vi "Team and Side.vi"(5 "Lado":enum16{"Esquerdo", "Direito"}(ring) caption="Enum", 7 "Time":enum16{"Azul", "Amarelo"}(ring) caption="Enum", 8 "Enemy state and balls":T2, 9 "IA_State":T12, 10 "Game Status":T18 {"Time" format="%<%.3X %x>T"; "Blue Timeout Remaining" format="%<%M:%S>t"; "Yellow Timeout Remaining" format="%<%M:%S>t"; "Time Left" format="%<%M:%S>t"}, 11 "Field State Input":T13 {"Detection Frame Out"."robots_blue"."height" format="%+4.3f"; "Detection Frame Out"."robots_blue"."pixel_y" format="%+4.3f"; "Detection Frame Out"."robots_blue"."pixel_x" format="%+4.3f"; "Detection Frame Out"."robots_blue"."orientation" format="%+4.3f"; "Detection Frame Out"."robots_blue"."y" format="%+4.3f"; "Detection Frame Out"."robots_blue"."confidence" format="%4.3f"; "Detection Frame Out"."robots_blue"."x" format="%+4.3f"; "Detection Frame Out"."robots_yellow"."height" format="%+4.3f"; "Detection Frame Out"."robots_yellow"."pixel_y" format="%+4.3f"; "Detection Frame Out"."robots_yellow"."pixel_x" format="%+4.3f"; "Detection Frame Out"."robots_yellow"."orientation" format="%+4.3f"; "Detection Frame Out"."robots_yellow"."y" format="%+4.3f"; "Detection Frame Out"."robots_yellow"."confidence" format="%4.3f"; "Detection Frame Out"."robots_yellow"."x" format="%+4.3f"}) -> (3 "IA State":T7={"our_robots"=[], "enemy_robots"=[], "balls"=[], "geometry"={"line_width"=0, "field_length"=0, "field_width"=0, "boundary_width"=0, "referee_width"=0, "goal_width"=0, "goal_depth"=0, "goal_wall_width"=0, "center_circle_radius"=0, "defense_radius"=0, "defense_stretch"=0, "free_kick_from_defense_dist"=0, "penalty_spot_from_field_line_dist"=0, "penalty_line_from_spot_dist"=0}, "IA Judge"={"stage"="", "command"="", "our_goalie_id"=0.0, "enemy_goalie_id"=0.0, "command enum"=enum."Halt", "Time"=enum."Azul"}, "Received Timestamp"=timestamp(0 s since 1904-01-01), "Events"={"Touch"=FALSE, "Ball out"=FALSE, "id touch"=0.0, "Ball out of \nVision"=FALSE, "Ball inside \nGoalie area"=FALSE, "Robot not responding"=FALSE, "Robots responding status"=[1.0, 1.0, 1.0, 1.0, 1.0, 1.0], "Enemy Ball \nPossession"=FALSE, "Pass State"=FALSE, "id end of pass"=0.0, "Kick"=FALSE, "Id ini Possession"=0.0, "Ball Possesion"=FALSE, "Id Possesion"=0.0}})   [LabVIEW 2017]
uses:
  SSL Referee Game Status.ctl
  AI Input.ctl
  AI Robot.ctl
  Intel/Functions Enum.ctl
  Intel/AttackerStates.ctl
  AI Ball.ctl
  Field Size.ctl
  AI Judge.ctl
  Intel/Command Enum.ctl
  Util/Events/Events.ctl
  SSL/SSL Field State.ctl
  SSL Detection Frame.ctl
  SSL Detection Robot.ctl
  <vilib>/Analysis/Matrix/Datatypes/RealMatrix.ctl
  SSL Detection Ball.ctl
  <vilib>/Analysis/Matrix/NI_Matrix.lvlib
panel:
  in  "enemy_robots":T3[](array[typedef])
  in  "?":T6
  in  "?":T6
  in  "output cluster":T7={"our_robots"=[], "enemy_robots"=[], "balls"=[], "geometry"={"line_width"=0, "field_length"=0, "field_width"=0, "boundary_width"=0, "referee_width"=0, "goal_width"=0, "goal_depth"=0, "goal_wall_width"=0, "center_circle_radius"=0, "defense_radius"=0, "defense_stretch"=0, "free_kick_from_defense_dist"=0, "penalty_spot_from_field_line_dist"=0, "penalty_line_from_spot_dist"=0}, "IA Judge"={"stage"="", "command"="", "our_goalie_id"=0.0, "enemy_goalie_id"=0.0, "command enum"=enum."Halt", "Time"=enum."Azul"}, "Received Timestamp"=timestamp(0 s since 1904-01-01), "Events"={"Touch"=FALSE, "Ball out"=FALSE, "id touch"=0.0, "Ball out of \nVision"=FALSE, "Ball inside \nGoalie area"=FALSE, "Robot not responding"=FALSE, "Robots responding status"=[1.0, 1.0, 1.0, 1.0, 1.0, 1.0], "Enemy Ball \nPossession"=FALSE, "Pass State"=FALSE, "id end of pass"=0.0, "Kick"=FALSE, "Id ini Possession"=0.0, "Ball Possesion"=FALSE, "Id Possesion"=0.0}}
  # "Score"
  # "Red Cards"
  # "Yellow Cards"
  # "Timeouts Left"
  # "Timeout Remaining"
  # "Goalie ID"
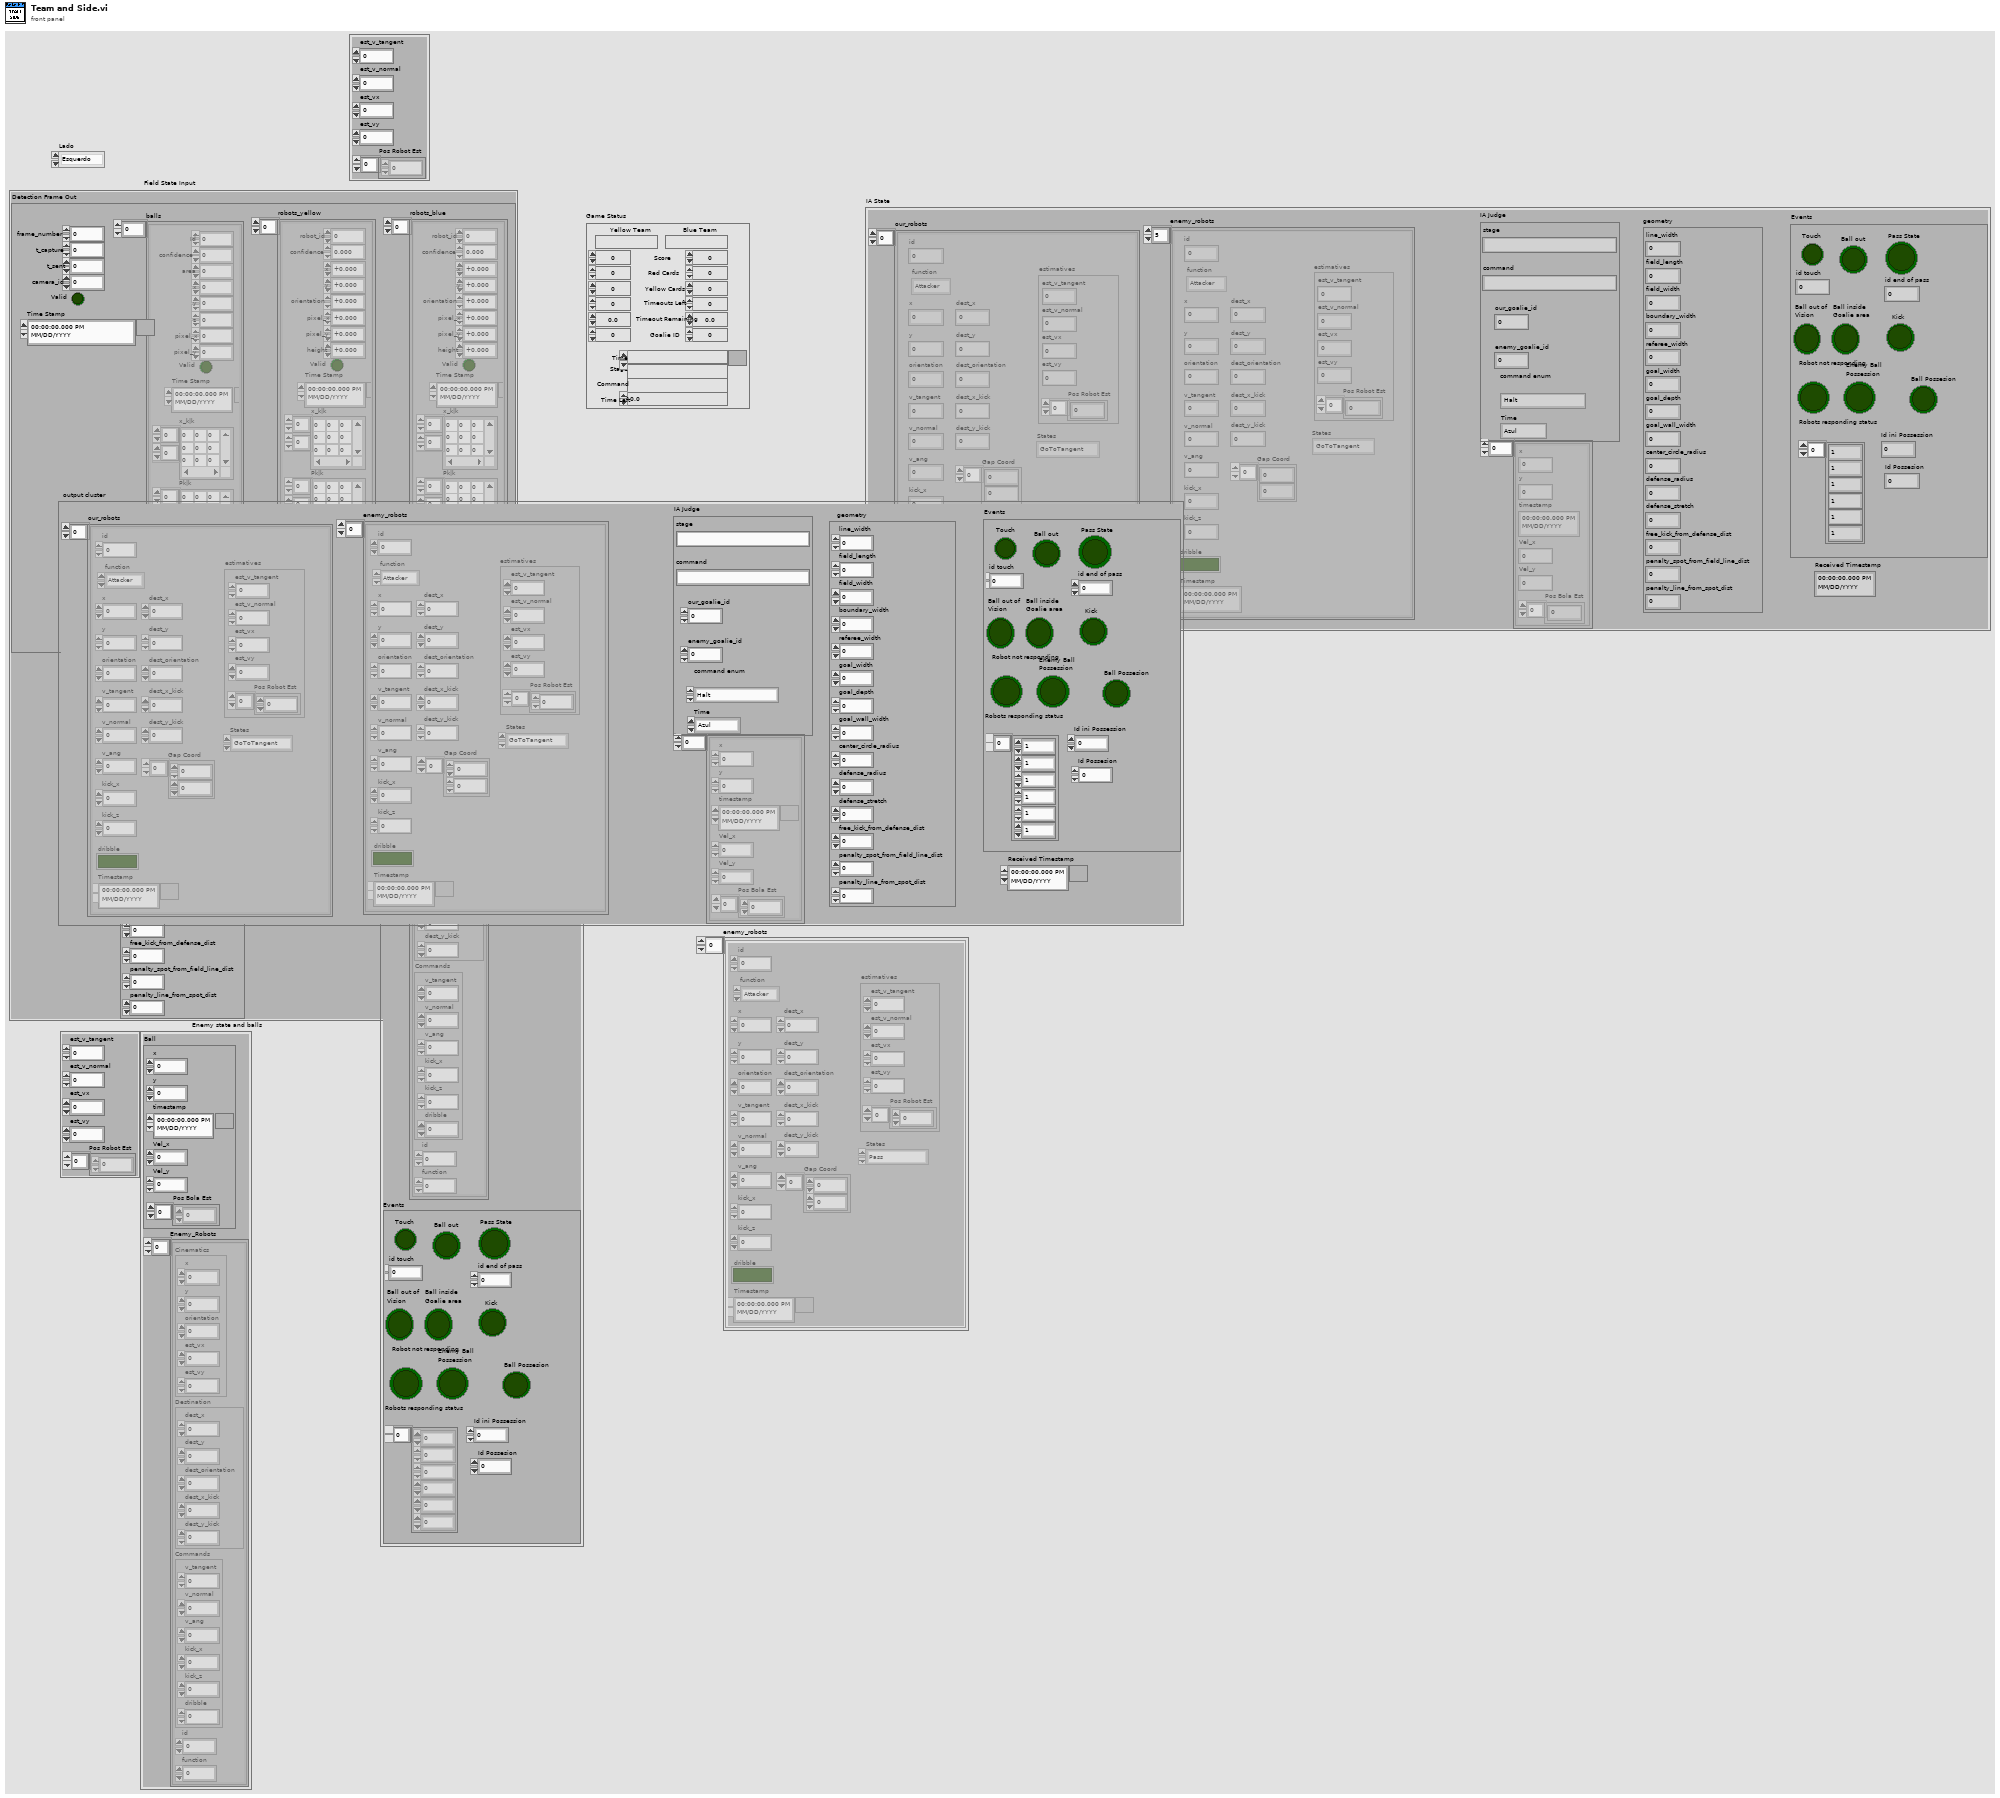
[diagram p1: front panel]
types:
  T1 = typedef "AI Ball.ctl" = cluster{"x":dbl, "y":dbl, "timestamp":timestamp, "Vel_x":dbl, "Vel_y":dbl, "Pos Bola Est":dbl[]}
  T2 = cluster{"Ball":T1, "Enemy_Robots":cluster{"Cinematics":cluster{"x":dbl, "y":dbl, "orientation":dbl, "est_vx":dbl, "est_vy":dbl}, "Destination":cluster{"dest_x":dbl, "dest_y":dbl, "dest_orientation":dbl, "dest_x_kick":dbl, "dest_y_kick":dbl}, "Commands":cluster{"v_tangent":dbl, "v_normal":dbl, "v_ang":dbl, "kick_x":dbl, "kick_z":dbl, "dribble":u32}, "id":u32, "function":u32}[]}
  T3 = typedef "AI Robot.ctl" = cluster{"id":u32, "function":T4, "x":dbl, "y":dbl, "orientation":dbl, "v_tangent":dbl, "v_normal":dbl, "v_ang":dbl, "kick_x":dbl, "kick_z":dbl, "dribble":bool, "Timestamp":timestamp, "dest_x":dbl, "dest_y":dbl, "dest_orientation":dbl, "estimatives":cluster{"est_v_tangent":dbl, "est_v_normal":dbl, "est_vx":dbl, "est_vy":dbl, "Pos Robot Est":dbl[]}, "dest_x_kick":dbl, "dest_y_kick":dbl, "Gap Coord":dbl[], "States":T5}
  T4 = typedef "Functions Enum.ctl" = enum16{"Attacker", "Goalie", "Defender", "Striker", "Goto 0", "Dummy", "Kicker", "ZigZag"}
  T5 = typedef "AttackerStates.ctl" = enum16{"Pass", "GoToTangent", "BallGetting", "GoToKick", ""}
  T6 = cluster{"est_v_tangent":dbl, "est_v_normal":dbl, "est_vx":dbl, "est_vy":dbl, "Pos Robot Est":dbl[]}
  T7 = typedef "AI Input.ctl" = cluster{"our_robots":T3[], "enemy_robots":T3[], "balls":T1[], "geometry":T8, "IA Judge":T9, "Received Timestamp":timestamp, "Events":T11}
  T8 = typedef "Field Size.ctl" = cluster{"line_width":u32, "field_length":u32, "field_width":u32, "boundary_width":u32, "referee_width":u32, "goal_width":u32, "goal_depth":u32, "goal_wall_width":u32, "center_circle_radius":u32, "defense_radius":u32, "defense_stretch":u32, "free_kick_from_defense_dist":u32, "penalty_spot_from_field_line_dist":u32, "penalty_line_from_spot_dist":u32}
  T9 = typedef "AI Judge.ctl" = cluster{"stage":string, "command":string, "our_goalie_id":dbl, "enemy_goalie_id":dbl, "command enum":T10, "Time":enum16{"Azul", "Amarelo"}}
  T10 = typedef "Command Enum.ctl" = enum16{"Halt", "Stop", "Force Start", "PKA Normal Start", "Prepare Kickoff Ally", "PKE Normal Start", "Prepare Kickoff Enemy", "Prepare Penalty Ally", "PPA Normal Start", "Prepare Penalty Enemy", "PPE Normal Start", "Direct Free Enemy", "Direct Free Ally", "Indirect Free Enemy", "Indirect Free Ally", "Timeout Enemy", "Timeout Ally", "Goal Enemy", "Goal Ally", "Ball Placement Enemy", "Ball Placement Ally", "Normal Half Time", "Extra Time Break", "Extra Half Time", "None", "Post Game"}
  T11 = typedef "Events.ctl" = cluster{"Touch":bool, "Ball out":bool, "id touch":dbl, "Ball out of \nVision":bool, "Ball inside \nGoalie area":bool, "Robot not responding":bool, "Robots responding status":dbl[], "Enemy Ball \nPossession":bool, "Pass State":bool, "id end of pass":dbl, "Kick":bool, "Id ini Possession":dbl, "Ball Possesion":bool, "Id Possesion":dbl}
  T12 = cluster{"Our_Robots":cluster{"Cinematics":cluster{"x":dbl, "y":dbl, "orientation":dbl, "est_vx":dbl, "est_vy":dbl}, "Destination":cluster{"dest_x":dbl, "dest_y":dbl, "dest_orientation":dbl, "dest_x_kick":dbl, "dest_y_kick":dbl}, "Commands":cluster{"v_tangent":dbl, "v_normal":dbl, "v_ang":dbl, "kick_x":dbl, "kick_z":dbl, "dribble":u32}, "id":u32, "function":u32}[], "Events":T11}
  T13 = typedef "SSL Field State.ctl" = cluster{"Detection Frame Out":T14, "Field Size Out":cluster{"line_width":u32, "field_length":u32, "field_width":u32, "boundary_width":u32, "referee_width":u32, "goal_width":u32, "goal_depth":u32, "goal_wall_width":u32, "center_circle_radius":u32, "defense_radius":u32, "defense_stretch":u32, "free_kick_from_defense_dist":u32, "penalty_spot_from_field_line_dist":u32, "penalty_line_from_spot_dist":u32}, "Received Time Stamp":timestamp}
  T14 = typedef "SSL Detection Frame.ctl" = cluster{"frame_number":u32, "t_capture":dbl, "t_sent":dbl, "camera_id":u32, "robots_yellow":T15[], "robots_blue":T15[], "balls":T17[], "Valid":bool, "Time Stamp":timestamp}
  T15 = typedef "SSL Detection Robot.ctl" = cluster{"x":sgl, "robot_id":u32, "confidence":sgl, "y":sgl, "orientation":sgl, "pixel_x":sgl, "pixel_y":sgl, "height":sgl, "Valid":bool, "Time Stamp":timestamp, "x_k|k":T16, "Pk|k":T16, "Previous Time Stamp":timestamp, "R":T16}
  T16 = typedef "NI_Matrix.lvlib/RealMatrix.ctl" = dbl[][]
  T17 = typedef "SSL Detection Ball.ctl" = cluster{"x":sgl, "area":u32, "confidence":sgl, "y":sgl, "z":sgl, "pixel_x":sgl, "pixel_y":sgl, "Valid":bool, "Time Stamp":timestamp, "x_k|k":T16, "Pk|k":T16, "Id":u32, "Previous Time Stamp":timestamp, "R":T16}
  T18 = typedef "SSL Referee Game Status.ctl" = cluster{"Stage":string, "Command":string, "Time Left":dbl, "Yellow Team":string, "Blue Team":string, "Yellow Score":u32, "Blue Score":u32, "Yellow Red Cards":u32, "Blue Red Cards":u32, "Yellow Yellow Cards":u32, "Blue Yellow Cards":u32, "Yellow Timeouts Left":u32, "Blue Timeouts Left":u32, "Yellow Timeout Remaining":dbl, "Blue Timeout Remaining":dbl, "Yellow Goalie Id":u32, "Blue Goalie Id":u32, "Time":timestamp}
  T19 = cluster{"Cinematics":cluster{"x":dbl, "y":dbl, "orientation":dbl, "est_vx":dbl, "est_vy":dbl}, "Destination":cluster{"dest_x":dbl, "dest_y":dbl, "dest_orientation":dbl, "dest_x_kick":dbl, "dest_y_kick":dbl}, "Commands":cluster{"v_tangent":dbl, "v_normal":dbl, "v_ang":dbl, "kick_x":dbl, "kick_z":dbl, "dribble":u32}, "id":u32, "function":u32}[]
  T20 = cluster{"line_width":u32, "field_length":u32, "field_width":u32, "boundary_width":u32, "referee_width":u32, "goal_width":u32, "goal_depth":u32, "goal_wall_width":u32, "center_circle_radius":u32, "defense_radius":u32, "defense_stretch":u32, "free_kick_from_defense_dist":u32, "penalty_spot_from_field_line_dist":u32, "penalty_line_from_spot_dist":u32}
  T21 = cluster{"x":dbl, "y":dbl, "orientation":dbl, "est_vx":dbl, "est_vy":dbl}
  T22 = cluster{"dest_x":dbl, "dest_y":dbl, "dest_orientation":dbl, "dest_x_kick":dbl, "dest_y_kick":dbl}
  T23 = cluster{"v_tangent":dbl, "v_normal":dbl, "v_ang":dbl, "kick_x":dbl, "kick_z":dbl, "dribble":u32}
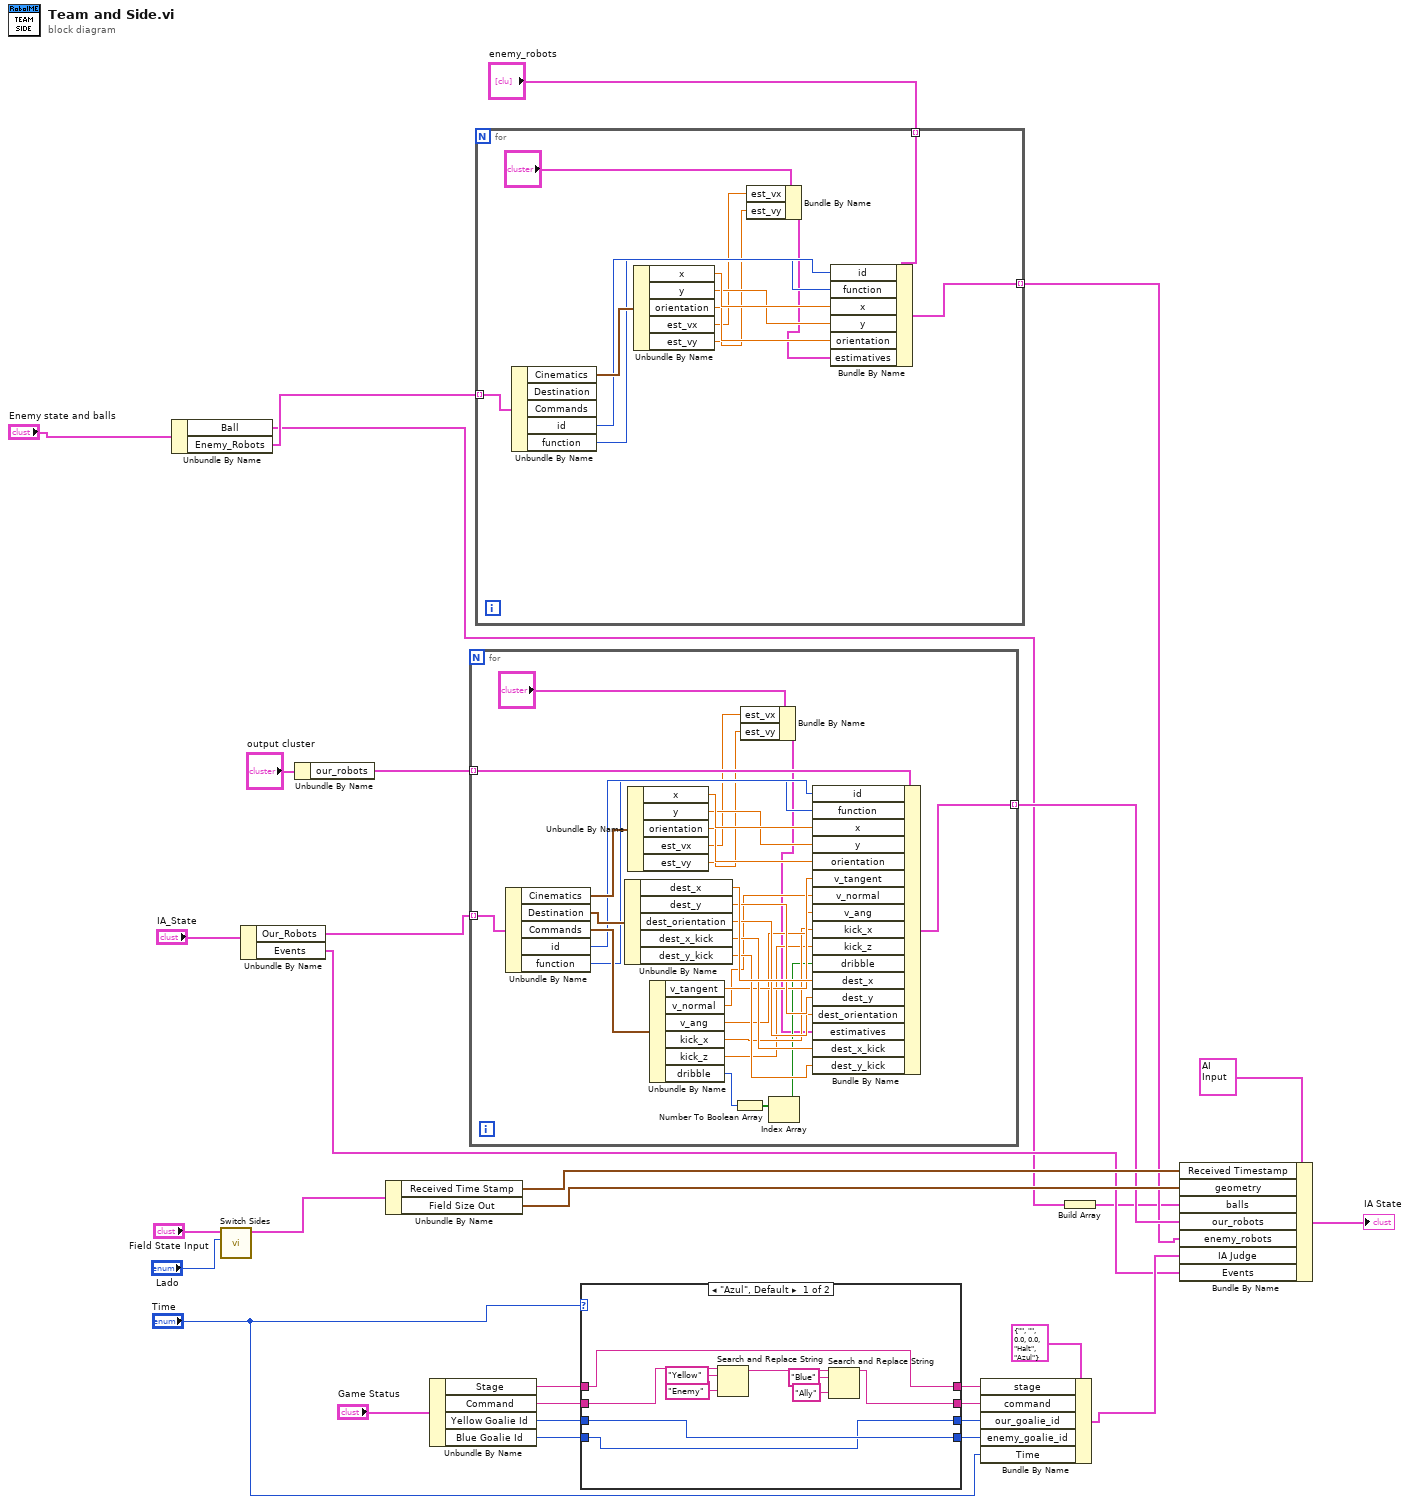
[diagram p0: block diagram]
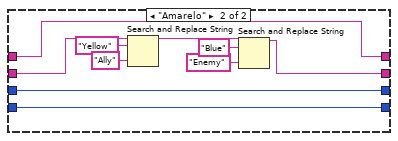
[diagram p2: hidden frame]
diagram:
  n1 = Unbundle By Name("Enemy state and balls") -> ("Ball"=w1:T1, "Enemy_Robots"=w3:T19)
  n2 = call "Switch Sides.vi"("Lado"="Lado", "Field State Input"="Field State Input") -> ("Field State Side Mirrored"=w30:T13)  [unwired: 9 in]
  n3 = Unbundle By Name("IA_State") -> ("Our_Robots"=w11:T19, "Events"=w7:T11)
  n4 = Unbundle By Name("output cluster") -> ("our_robots"=w9:T3[])
  n5 = Unbundle By Name(w30) -> ("Received Time Stamp"=w15:timestamp, "Field Size Out"=w18:T20)
  n6 = Unbundle By Name("Game Status") -> ("Stage"=w24:string, "Command"=w23:string, "Yellow Goalie Id"=w27:u32, "Blue Goalie Id"=w26:u32)
  n7 = for {
    tunnel: w11 -> [w59] mode=indexing
    tunnel: w9 -> [w57] mode=indexing
    tunnel: [w56] -> w8 mode=indexing
    n8 = Unbundle By Name(w59) -> ("Cinematics"=w58:T21, "Destination"=w55:T22, "Commands"=w54:T23, "id"=w37:u32, "function"=w36:u32)
    n9 = Unbundle By Name(w55) -> ("dest_x"=w50:dbl, "dest_y"=w49:dbl, "dest_orientation"=w48:dbl, "dest_x_kick"=w47:dbl, "dest_y_kick"=w46:dbl)
    n10 = Unbundle By Name(w58) -> ("x"=w53:dbl, "y"=w52:dbl, "orientation"=w51:dbl, "est_vx"=w34:dbl, "est_vy"=w33:dbl)
    n11 = Unbundle By Name(w54) -> ("v_tangent"=w45:dbl, "v_normal"=w44:dbl, "v_ang"=w43:dbl, "kick_x"=w42:dbl, "kick_z"=w41:dbl, "dribble"=w40:u32)
    n12 = Number To Boolean Array(number=w40) -> (Boolean array=w38:bool[])
    n13 = Bundle By Name(cluster="?", "est_vx"=w34, "est_vy"=w33) -> (w32:T6)
    n14 = Index Array(array=w38) -> (element=w39:bool)  [unwired: 1 in]
    n15 = Bundle By Name(cluster=w57, "id"=w37, "function"=w36, "x"=w53, "y"=w52, "orientation"=w51, "v_tangent"=w45, "v_normal"=w44, "v_ang"=w43, "kick_x"=w42, "kick_z"=w41, "dribble"=w39, "dest_x"=w50, "dest_y"=w49, "dest_orientation"=w48, "estimatives"=w32, "dest_x_kick"=w47, "dest_y_kick"=w46) -> (w56:T3)
  }
  n16 = for {
    tunnel: w3 -> [w72] mode=indexing
    tunnel: [w70] -> w5 mode=indexing
    tunnel: "enemy_robots" -> [w60] mode=indexing
    n17 = Unbundle By Name(w72) -> ("Cinematics"=w71:T21, "id"=w66:u32, "function"=w65:u32)  [unwired: 2 out]
    n18 = Unbundle By Name(w71) -> ("x"=w69:dbl, "y"=w68:dbl, "orientation"=w67:dbl, "est_vx"=w63:dbl, "est_vy"=w62:dbl)
    n19 = Bundle By Name(cluster="?", "est_vx"=w63, "est_vy"=w62) -> (w61:T6)
    n20 = Bundle By Name(cluster=w60, "id"=w66, "function"=w65, "x"=w69, "y"=w68, "orientation"=w67, "estimatives"=w61) -> (w70:T3)
  }
  n21 = case shown="\"Azul\", Default" "Time" {
    tunnel: w27 -> [w82 w92]
    tunnel: w26 -> [w81 w91]
    tunnel: [w82 w91] -> w21
    tunnel: [w81 w92] -> w22
    tunnel: w24 -> [w73 w90]
    tunnel: w23 -> [w75 w89]
    tunnel: [w73 w90] -> w20
    tunnel: [w74 w83] -> w19
    frame "Azul", Default {
      n22 = Search and Replace String(input string=w75, search string="Yellow", replace string="Enemy" ("replace string (\"\")")) -> (result string=w80:string)  [unwired: 5 in, 3 out]
      n23 = Search and Replace String(input string=w80, search string="Blue", replace string="Ally" ("replace string (\"\")")) -> (result string=w74:string)  [unwired: 5 in, 3 out]
    }
    frame "Amarelo" {
      n24 = Search and Replace String(input string=w89, search string="Yellow", replace string="Ally" ("replace string (\"\")")) -> (result string=w84:string)  [unwired: 5 in, 3 out]
      n25 = Search and Replace String(input string=w84, search string="Blue", replace string="Enemy" ("replace string (\"\")")) -> (result string=w83:string)  [unwired: 5 in, 3 out]
    }
  }
  n26 = Bundle By Name(cluster=T9 {"stage"="", "command"="", "our_goalie_id"=0.0, "enemy_goalie_id"=0.0, "command enum"=enum."Halt", "Time"=enum."Azul"} ("IA Judge"), "stage"=w20, "command"=w19, "our_goalie_id"=w22, "enemy_goalie_id"=w21, "Time"="Time") -> (w14:T9)
  n27 = Build Array(w1) -> (w2:T1[])
  n28 = Bundle By Name(cluster=T7 {"our_robots"=[], "enemy_robots"=[], "balls"=[], "geometry"={"line_width"=0, "field_length"=0, "field_width"=0, "boundary_width"=0, "referee_width"=0, "goal_width"=0, "goal_depth"=0, "goal_wall_width"=0, "center_circle_radius"=0, "defense_radius"=0, "defense_stretch"=0, "free_kick_from_defense_dist"=0, "penalty_spot_from_field_line_dist"=0, "penalty_line_from_spot_dist"=0}, "IA Judge"={"stage"="", "command"="", "our_goalie_id"=0.0, "enemy_goalie_id"=0.0, "command enum"=enum."Halt", "Time"=enum."Azul"}, "Received Timestamp"=timestamp(0 s since 1904-01-01), "Events"={"Touch"=FALSE, "Ball out"=FALSE, "id touch"=0.0, "Ball out of \nVision"=FALSE, "Ball inside \nGoalie area"=FALSE, "Robot not responding"=FALSE, "Robots responding status"=[1.0, 1.0, 1.0, 1.0, 1.0, 1.0], "Enemy Ball \nPossession"=FALSE, "Pass State"=FALSE, "id end of pass"=0.0, "Kick"=FALSE, "Id ini Possession"=0.0, "Ball Possesion"=FALSE, "Id Possesion"=0.0}} ("Detection Frame"), "Received Timestamp"=w15, "geometry"=w18, "balls"=w2, "our_robots"=w8, "enemy_robots"=w5, "IA Judge"=w14, "Events"=w7) -> (→"IA State":T7)
